vi "Self-Test.vi"(8 "error in (no error)":errorcluster, 11 "DPO4104 in":refnum<class "DPO4104.lvclass">) -> (0 "error out":errorcluster, 2 "Self-Test Passed? (T:Yes)":bool, 3 "DPO4104 out":refnum<class "DPO4104.lvclass">)   [LabVIEW 2018, in "DPO4104.lvlib" / "DPO4104.lvclass"]
doc: "This Override method is used to call the Self-Test function of the Oscope instrument. The boolean output 'Self-Test Passed? (T:Yes)' carries out the Self-Test result."
uses:
  DPO4104.lvclass
  <instrlib>/Tektronix DPO MSO 2000 4000 Series/Tektronix DPO MSO 2000 4000 Series.lvlib
  PPLs/Oscilloscope/Parent/Oscilloscope.lvlibp/Oscilloscope.lvclass
  C:/Projects/LabVIEW/PPLs/Oscilloscope/Parent/Oscilloscope.lvlibp/Oscilloscope.lvclass
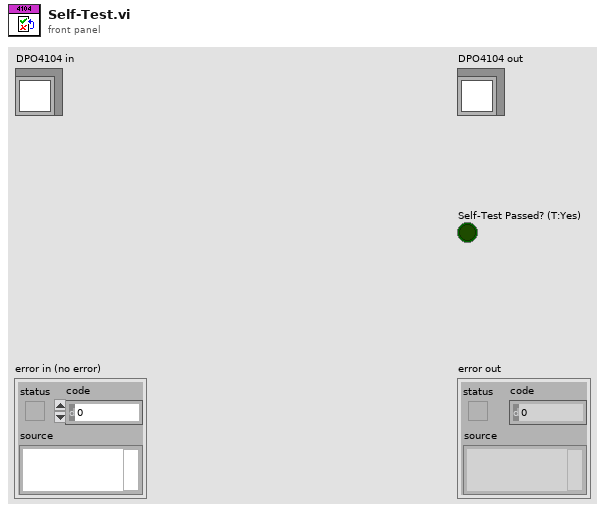
[diagram p1: front panel]
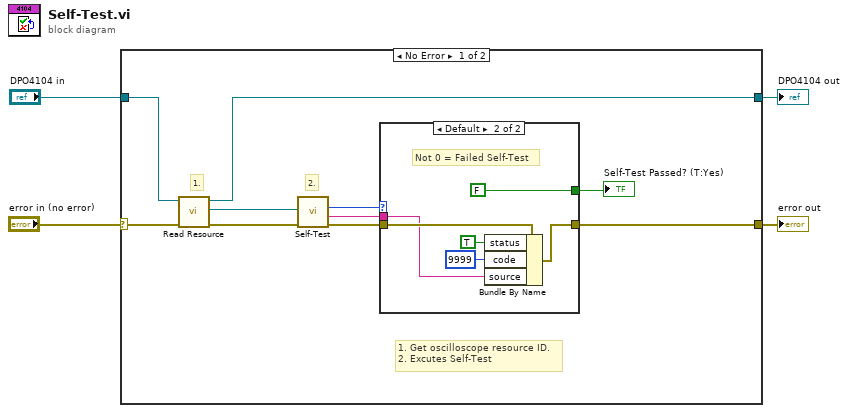
[diagram p0: block diagram]
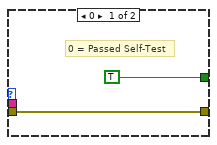
[diagram p2: hidden frame]
diagram:
  n1 = case shown="No Error" "error in (no error)" {
    selector: "error in (no error)" -> [w9 w24]
    tunnel: [w6 w23] -> w4
    tunnel: "DPO4104 in" -> [w11 w23]
    tunnel: [w10 w24] -> w2
    frame No Error {
      # "1. Get oscilloscope resource ID.\n2. Excutes Self-Test"
      # "2."
      # "1."
      n2 = call "Read Resource.vi"("error in (no error)"=w9, "Oscilloscope in"=w11) -> ("error out"=w5:errorcluster, "Resource"=w7:refnum<visa-resource-name>, "Oscilloscope out"=w6:refnum<class "DPO4104.lvclass">)  [unwired: 7 in]
      n3 = call <instrlib>:"Self-Test.vi"("error in (no error)"=w5, "VISA resource name"=w7) -> ("error out"=w13:errorcluster, "Self-Test Result Message"=w12:string, "Self-Test Result Code"=w14:i32)  [unwired: 6 in, 1 out]
      n4 = case shown="Default" w14 {
        tunnel: w13 -> [w16 w21]
        tunnel: w12 -> [_ w17]
        tunnel: [w16 w20] -> w10
        tunnel: [TRUE FALSE] -> w8
        frame 0 {
          # "0 = Passed Self-Test"
        }
        frame Default {
          # "Not 0 = Failed Self-Test"
          n5 = Bundle By Name(cluster=w21, "status"=TRUE, "code"=9999, "source"=w17) -> (w20:errorcluster)
        }
      }
      "Self-Test Passed? (T:Yes)" <- w8
    }
    frame Error {
    }
  }
  "error out" <- w2
  "DPO4104 out" <- w4
